vi "nanomsg_send.vi"(2 "error in":errorcluster, 3 "no block? (F)":bool, 4 "data":string, 5 "socket in":refnum<class "nanomsg_socket.lvclass">) -> (0 "error out":errorcluster, 1 "socket out":refnum<class "nanomsg_socket.lvclass">)   [LabVIEW 2014, in "nanomsg.lvlib" / "nanomsg_socket.lvclass"]
doc: "Add the binary string <b>data</b> (the NULL value \\0 is permitted) to the output queue of the socket <b>socket in</b>.\n\nIf <b>no block?</b> is True, the function returns immediately regardless of whether the message entered the queue successfully (not recommended).\n\nNote that when this call returns the message will likely <b>not have been sent yet</b> as it has only been placed in the queue for sending."
uses:
  nanomsg_socket.lvclass
  nanomsg_socket.lvclass/nanomsg_socket.ctl
  <vilib>/Utility/error.llb/Error Cluster From Error Code.vi
  nanomsg.lvlib
panel:
  # "NN"
  # "labview"
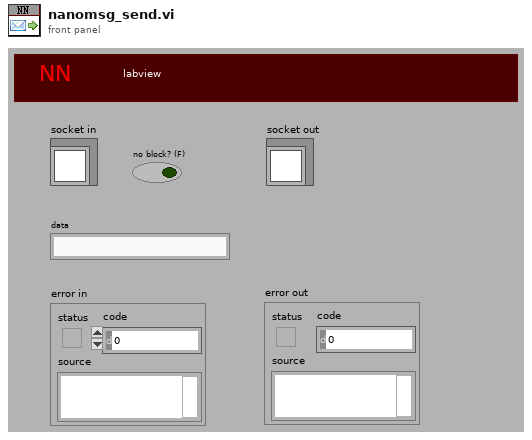
[diagram p1: front panel]
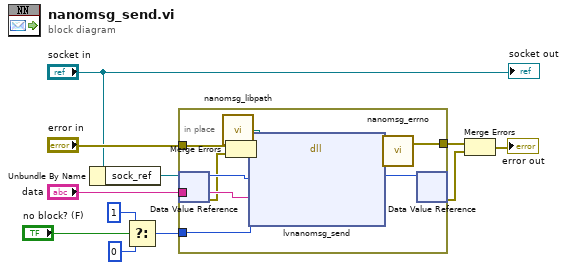
[diagram p0: block diagram]
diagram:
  n1 = Unbundle By Name("socket in") -> ("sock_ref"=w3:refnum<data-value>)
  n2 = Select(t=1 ("flags"), s="no block? (F)", f=0 ("flags")) -> (s? t:f=w5:i32)
  n3 = in-place {
    in-place-border: "error in" -> [w22]
    in-place-border: "data" -> [w21]
    in-place-border: [w18] -> w9
    in-place-border: w5 -> [w17]
    n4 = in-place-dvr #1(w3) -> (w16:u64, w12:errorcluster)
    n5 = call "nanomsg_libpath.vi"() -> ("path"=w14:path)
    n6 = Merge Errors(w22, w12) -> (w13:errorcluster)
    n7 = dll-call lib="?" fn="lvnanomsg_send" ("zmq_labview.dll:lvzmq_socket")(path in=w14, error in=w13, "sock_obj"=w16, "data"=w21, "flags"=w17) -> (error out=w20:errorcluster, "return type"=w19:i32, "sock_obj"=w15:u64)  [unwired: 3 in, 1 out]
    n8 = call "nanomsg_errno.vi"("retval"=w19, "error in"=w20) -> ("error out"=w18:errorcluster)  [unwired: 1 out]
    n9 = in-place-dvr #1(w15) -> (w1:errorcluster)  [unwired: 1 out]
  }
  n10 = Merge Errors(w9, w1) -> (→"error out":errorcluster)
  "socket out" <- "socket in"
